vi "TEMPLATE_Regular_Return.vi"(8 "Error In":errorcluster, 11 "%TYPE% In":refnum<class "LQIdentity.lvclass">) -> (0 "Error Out":errorcluster, 2 "Value":string, 3 "%TYPE% Out":refnum<class "LQIdentity.lvclass">)   [LabVIEW 2014, in "Template.lvlib" / "LQIdentity.lvclass"]
uses:
  LQIdentity.lvclass
  LQIdentity.lvclass/LQIdentity.ctl
  Template.lvlib
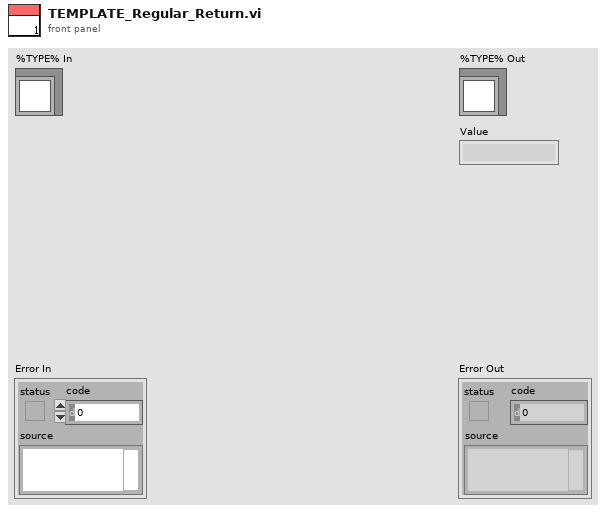
[diagram p1: front panel]
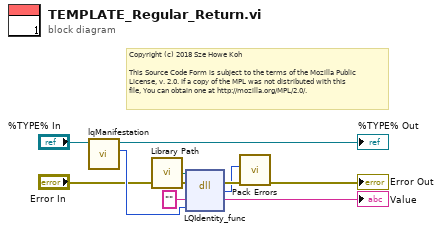
[diagram p0: block diagram]
diagram:
  # "Copyright (c) 2018 Sze Howe Koh\n\nThis Source Code Form is subject to the terms of the Mozilla Public\nLicense, v. 2.0. If a copy of the MPL was not distributed with this\nfile, You can obtain one at http://mozilla.org/MPL/2.0/."
  n1 = call "lqManifestation.vi"("LQIdentity in"="%TYPE% In") -> ("Manifestation"=w5:u64, "LQIdentity out"=→"%TYPE% Out":refnum<class "LQIdentity.lvclass">)  [unwired: 9 in]
  n2 = call "Library Path.vi"() -> ("Library Path"=w6:path)
  n3 = dll-call lib="?" fn="LQIdentity_func"(path in=w6, error in="Error In", "retVal"="", "_instance"=w5) -> (error out=w3:errorcluster, "errorCode"=w1:i32, "retVal"=→"Value":string)  [unwired: 2 in, 1 out]
  n4 = call "Pack Errors.vi"("Error In"=w3, "Error Code"=w1) -> ("Error Out"=→"Error Out":errorcluster)  [unwired: 9 in]
